vi "Linear Helicopter Model.vi"(9 "motor voltage gain":dbl=1.0, 10 "motor voltage 2":dbl, 11 "motor voltage 1":dbl) -> (3 "output":T1)   [LabVIEW 2014]
uses:
  <vilib>/Simulation/Implementation/Shared/SIMSCR Execution Mode.ctl
  <vilib>/Simulation/Scripting/Companion Diagram/SimConfigNode/SimParams.ctl
  <vilib>/Simulation/Scripting/Companion Diagram/SimConfigNode/_simSolvers.ctl
  <vilib>/Simulation/Param Hierarchy/Typedefs/SIMPH Param Control Actions.ctl
  <vilib>/Simulation/Implementation/Shared/NILVSim_ParamChanged.vi
  <vilib>/Simulation/Implementation/Shared/NILVSIM_BeginStep.vi
  <vilib>/Simulation/ContinuousLinear/Implementation/NILVSim State Space.llb/SIM State Space Distributor (MIMO).vi
  <vilib>/Simulation/ContinuousLinear/Implementation/NILVSim State Space.llb/SIM State Space Collector (MIMO).vi
  <vilib>/Simulation/Implementation/Shared/NILVSim_Manager.vi
  <vilib>/Utility/error.llb/Clear Errors.vi
  <vilib>/Simulation/Implementation/Shared/NILVSim_FinalizeModel.vi
  <vilib>/Simulation/Implementation/Shared/SIM Unbundle Sim Info.vi
  <vilib>/Simulation/Implementation/Shared/SIMSH Read Queue.vi
  <vilib>/Simulation/Implementation/Shared/NILVSim_Initialize.vi
  <vilib>/Simulation/Utility/Implementation/NILVSim Get Time and IsAcceptedStep.vi
  <vilib>/Simulation/Implementation/Shared/NILVSim_GetModelError.vi
  <vilib>/Simulation/Implementation/Shared/SIM SimErrorHandler.vi
  <vilib>/Simulation/Implementation/Shared/SIM Bundle Sim Info.vi
  <vilib>/Simulation/Scripting/Companion Diagram/SimConfigNode/SimDog.xnode
  <vilib>/Simulation/Implementation/XNodeFramework/SimXNode/SimX.xnode
  <vilib>/Simulation/ContinuousLinear/Implementation/NILVSim State Space.llb/SIM State Space (MIMO).vi
  <vilib>/Simulation/Implementation/Shared/NI_SIM_Implementation.lvlib
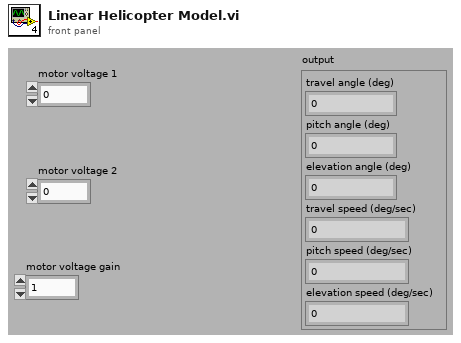
[diagram p1: front panel]
types:
  T1 = cluster{"travel angle (deg)":dbl, "pitch angle (deg)":dbl, "elevation angle (deg)":dbl, "travel speed (deg/sec)":dbl, "pitch speed (deg/sec)":dbl, "elevation speed (deg/sec)":dbl}
  T2 = cluster{"travel angle (deg)":dbl, "pitch angle (deg)":dbl, "elevation angle (deg)":dbl, "travel speed (deg per sec)":dbl, "pitch speed (deg per sec)":dbl, "elevation speed (deg per sec)":dbl}
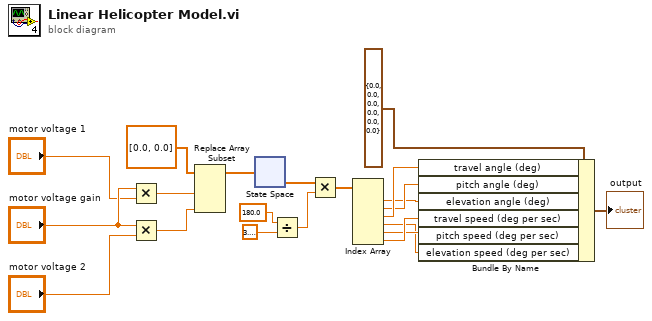
[diagram p0: block diagram]
diagram:
  n1 = Multiply ("Multiply 2")(x="motor voltage gain", y="motor voltage 1") -> (x*y=w2:dbl)
  n2 = Multiply ("Multiply 3")(x="motor voltage gain", y="motor voltage 2") -> (x*y=w1:dbl)
  n3 = Replace Array Subset(array=dbl[] [0.0, 0.0] ("Constant"), new element #1=w2, new element #2=w1) -> (w17:dbl[])  [unwired: 2 in]
  n4 = xnode ("State Space")("input u(t)"=w17) -> ("state x(t)"=w10:dbl[])  [unwired: 5 in, 1 out]
  n5 = Divide(x=180.0 ("Constant 2"), y=3.141592653589793 ("Constant 3")) -> (x/y=w6:dbl)
  n6 = Multiply(x=w10, y=w6) -> (x*y=w9:dbl[])
  n7 = Index Array(array=w9) -> (element #1=w12:dbl, element #2=w14:dbl, element #3=w16:dbl, element #4=w11:dbl, element #5=w13:dbl, element #6=w15:dbl)  [unwired: 6 in]
  n8 = Bundle By Name(cluster=T2 {"travel angle (deg)"=0.0, "pitch angle (deg)"=0.0, "elevation angle (deg)"=0.0, "travel speed (deg per sec)"=0.0, "pitch speed (deg per sec)"=0.0, "elevation speed (deg per sec)"=0.0} ("output 2"), "travel angle (deg)"=w16, "pitch angle (deg)"=w14, "elevation angle (deg)"=w12, "travel speed (deg per sec)"=w15, "pitch speed (deg per sec)"=w13, "elevation speed (deg per sec)"=w11) -> (→"output":T2)
